vi "Compile Data Replays.vi"(6 "Channel Descriptors in":T1, 7 "LoopName":string, 8 "error in (no error)":errorcluster, 9 "Custom Device Ref":T8 format="%.0x", 11 "Data Replays Refs":T8[](array[typedef]) format="%.0x") -> (0 "error out":errorcluster, 1 "DataReplayVoltages":T9[](array[typedef]), 3 "Data Replays":T10[](array[typedef]), 4 "Channel Descriptors out":T1)   [LabVIEW 2011, in "Engine Sim System Explorer.lvlib"]
uses:
  Engine Sim System Explorer.lvlib
  Shared/DataReplayConfig.ctl
  <vilib>/NI Veristand/Custom Device API/Custom Device Item Ref.ctl
  Shared/DataReplayVoltageConfig.ctl
  Shared/Channel Descriptors.ctl
  Shared/FPGA Write Descriptor.ctl
  Shared/InputChannelTypes.ctl
  <vilib>/rvi/DataTransferAndStorage/Container/Common/niFpgaDataTypeControl.ctl
  Shared/FPGA Read Descriptor.ctl
  Shared/OutputChannelTypes.ctl
  Shared/Status Chan Descriptor.ctl
  TypeDefs/DataReplayCtrlStringInfo.ctl
  TypeDefs/FPGA Mem Size.ctl
  Shared/Engine Simulation Global.vi
  <vilib>/NI Veristand/Custom Device API/Get Item Property (I32).vi
  <vilib>/NI Veristand/Custom Device API/Get Item Property (Boolean).vi
  <vilib>/NI Veristand/Custom Device API/Get Item Property (Double).vi
  <vilib>/NI Veristand/Custom Device API/Get Item Property (U16).vi
  Engine Simulation Shared.lvlib
  <vilib>/NI Veristand/Custom Device API/Custom Device API.lvlib
  <userlib>/AES/RT/AES RT.lvlib
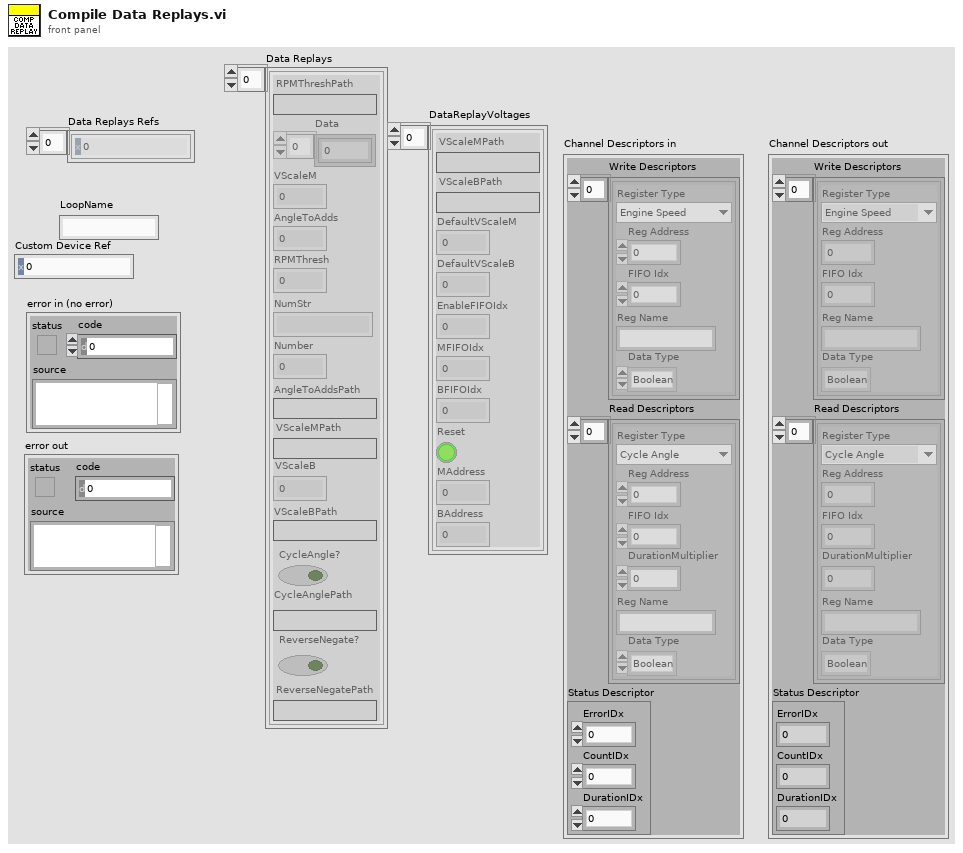
[diagram p1: front panel]
types:
  T1 = typedef "Engine Simulation Shared.lvlib/Channel Descriptors.ctl" = cluster{"Write Descriptors":T2[], "Read Descriptors":T5[], "Status Descriptor":T7}
  T2 = typedef "Engine Simulation Shared.lvlib/FPGA Write Descriptor.ctl" = cluster{"Register Type":T3, "Reg Address":u32, "FIFO Idx":i32, "Reg Name":string, "Data Type":T4}
  T3 = typedef "Engine Simulation Shared.lvlib/InputChannelTypes.ctl" = enum16{"Engine Speed", "Offset"}
  T4 = typedef "niFpgaDataTypeControl.ctl" = enum32{"Boolean", "I8", "I16", "I32", "I64", "U8", "U16", "U32", "U64", "FXP", "CustomControl"}
  T5 = typedef "Engine Simulation Shared.lvlib/FPGA Read Descriptor.ctl" = cluster{"Register Type":T6, "Reg Address":u32, "FIFO Idx":i32, "DurationMultiplier":dbl, "Reg Name":string, "Data Type":T4}
  T6 = typedef "Engine Simulation Shared.lvlib/OutputChannelTypes.ctl" = enum16{"Cycle Angle", "Crank Angle", "Time Duration", "Angle Duration", "Start Angle", "End Angle"}
  T7 = typedef "Engine Simulation Shared.lvlib/Status Chan Descriptor.ctl" = cluster{"ErrorIDx":i32, "CountIDx":i32, "DurationIDx":i32}
  T8 = typedef "Custom Device API.lvlib/Custom Device Item Ref.ctl" = u64
  T9 = typedef "Engine Simulation Shared.lvlib/DataReplayVoltageConfig.ctl" = cluster{"VScaleMPath":string, "VScaleBPath":string, "DefaultVScaleM":u32, "DefaultVScaleB":i32, "EnableFIFOIdx":i32, "MFIFOIdx":i32, "BFIFOIdx":i32, "Reset":bool, "MAddress":u32, "BAddress":u32}
  T10 = typedef "Engine Simulation Shared.lvlib/DataReplayConfig.ctl" = cluster{"RPMThreshPath":string, "Data":i16[], "VScaleM":u32, "AngleToAdds":u32, "RPMThresh":u64, "NumStr":string, "Number":i8, "AngleToAddsPath":string, "VScaleMPath":string, "VScaleB":i32, "VScaleBPath":string, "CycleAngle?":bool, "CycleAnglePath":string, "ReverseNegate?":bool, "ReverseNegatePath":string}
  T11 = typedef "Engine Sim System Explorer.lvlib/DataReplayCtrlStringInfo.ctl" = cluster{"LoopName":string, "ReplayName":string, "ReplayNumber":string}
  T12 = typedef "Engine Sim System Explorer.lvlib/FPGA Mem Size.ctl" = enum16{"32,768", "16,384", "8,192", "4,096", "2,048", "1024", "512", "256", "128"}
  T13 = typedef "Custom Device API.lvlib/Custom Device Item Info.ctl" = cluster{"Name":string, "Is Channel":bool, "GUID":string}
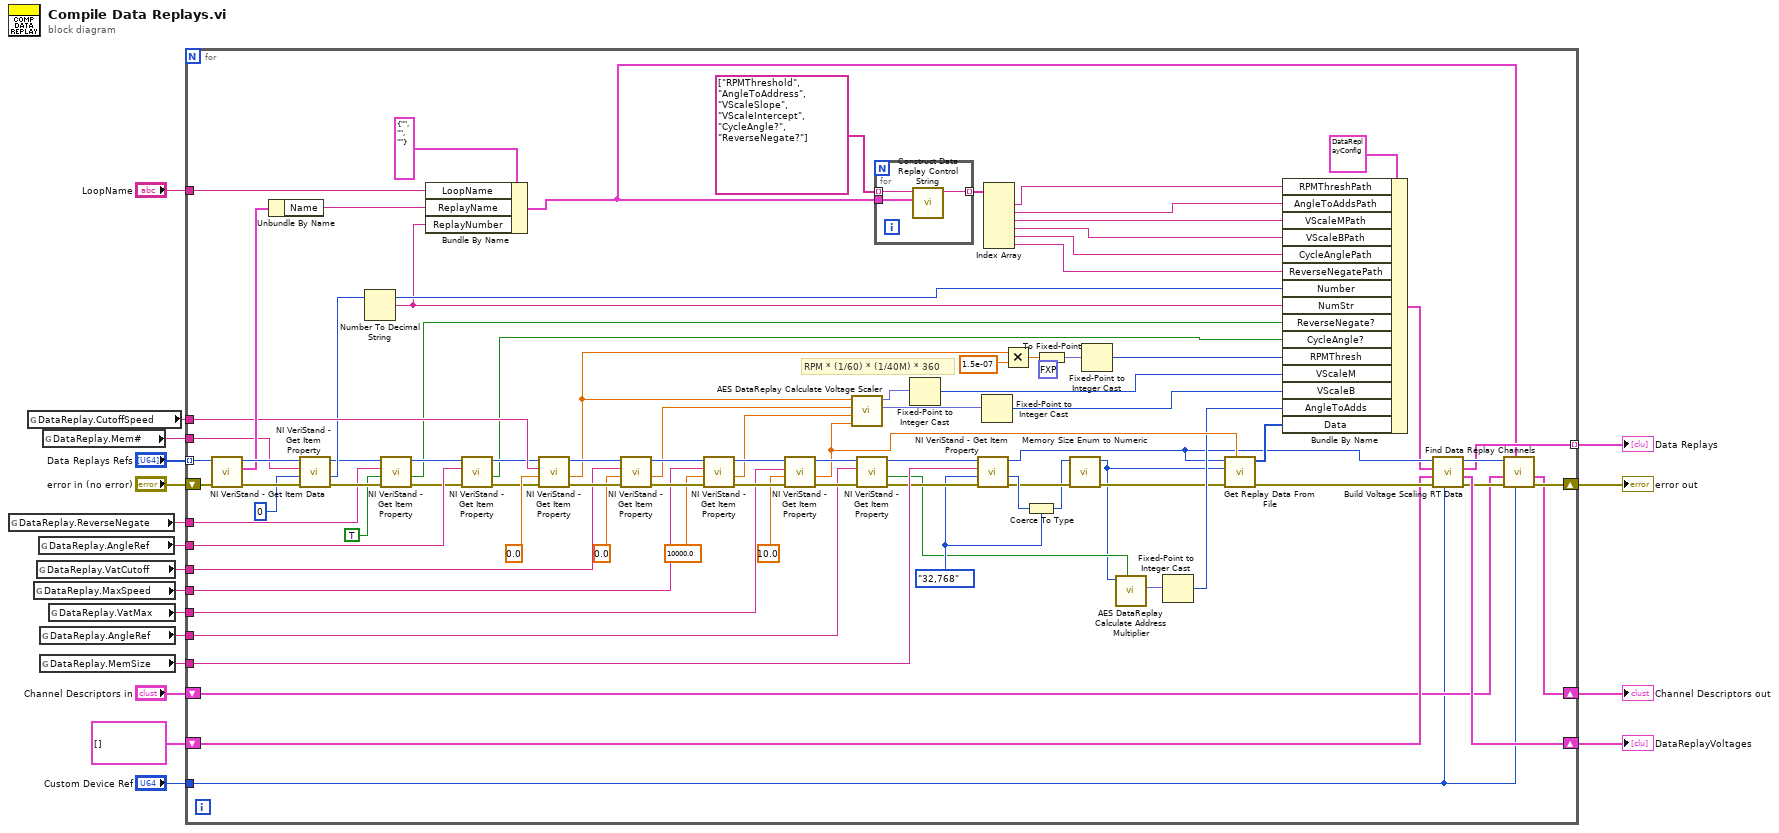
[diagram p0: block diagram]
diagram:
  n1 = global read "Engine Simulation Global.vi" "DataReplay.ReverseNegate"() -> (w6:string)
  n2 = global read "Engine Simulation Global.vi" "DataReplay.CutoffSpeed"() -> (w15:string)
  n3 = global read "Engine Simulation Global.vi" "DataReplay.MaxSpeed"() -> (w13:string)
  n4 = global read "Engine Simulation Global.vi" "DataReplay.VatCutoff"() -> (w14:string)
  n5 = global read "Engine Simulation Global.vi" "DataReplay.AngleRef"() -> (w7:string)
  n6 = global read "Engine Simulation Global.vi" "DataReplay.AngleRef"() -> (w11:string)
  n7 = global read "Engine Simulation Global.vi" "DataReplay.MemSize"() -> (w10:string)
  n8 = global read "Engine Simulation Global.vi" "DataReplay.Mem#"() -> (w16:string)
  n9 = global read "Engine Simulation Global.vi" "DataReplay.VatMax"() -> (w12:string)
  n10 = for {
    shift-right: [w30] -> w19
    shift-left: "error in (no error)" -> [w107]
    tunnel: "Data Replays Refs" -> [w104] mode=indexing
    tunnel: w16 -> [w101]
    tunnel: w15 -> [w92]
    tunnel: w14 -> [w91]
    tunnel: w13 -> [w90]
    tunnel: w12 -> [w89]
    tunnel: w11 -> [w80]
    tunnel: w10 -> [w78]
    tunnel: [w25] -> w9 mode=indexing
    tunnel: "LoopName" -> [w23]
    tunnel: w7 -> [w46]
    tunnel: w6 -> [w40]
    shift-right: [w35] -> w4
    shift-left: T9[] [] ("DataReplayVoltages") -> [w34]
    tunnel: "Custom Device Ref" -> [w26]
    shift-right: [w27] -> w1
    shift-left: "Channel Descriptors in" -> [w28]
    w62 = FPGA_Mem_Size."32,768" ("FPGA Memory Size")
    # "RPM * (1/60) * (1/40M) * 360"
    n11 = call <vilib>:"NI VeriStand - Get Item Data.vi"("error in (no error)"=w107, "Item Ref in"=w104) -> ("error out"=w105:errorcluster, "Item Info"=w102:T13, "Item Ref out"=w103:T8)  [unwired: 6 in, 1 out]
    n12 = Unbundle By Name(w102) -> ("Name"=w22:string)
    n13 = call-poly <vilib>:"NI VeriStand - Get Item Property.vi"("error in (no error)"=w105, "Default Value"=0, "Property Name"=w101, "Item Ref in"=w103) -> ("error out"=w96:errorcluster, "Value"=w68:i32, "Item Ref out"=w42:T8)  [unwired: 4 in, 1 out]
    n14 = Number To Decimal String(number=w68) -> (decimal integer string=w21:string)  [unwired: 1 in]
    n15 = call-poly <vilib>:"NI VeriStand - Get Item Property.vi"("error in (no error)"=w96, "Default Value"=TRUE, "Property Name"=w40, "Item Ref in"=w42) -> ("error out"=w43:errorcluster, "Value"=w38:bool, "Item Ref out"=w41:T8)  [unwired: 4 in, 1 out]
    n16 = Bundle By Name(cluster=T11 {"LoopName"="", "ReplayName"="", "ReplayNumber"=""} ("Control String Info"), "LoopName"=w23, "ReplayName"=w22, "ReplayNumber"=w21) -> (w20:T11)
    n17 = call-poly <vilib>:"NI VeriStand - Get Item Property.vi"("error in (no error)"=w43, "Property Name"=w46, "Item Ref in"=w41) -> ("error out"=w48:errorcluster, "Value"=w45:bool, "Item Ref out"=w47:T8)  [unwired: 5 in, 1 out]
    n18 = call-poly <vilib>:"NI VeriStand - Get Item Property.vi"("error in (no error)"=w48, "Default Value"=0.0, "Property Name"=w92, "Item Ref in"=w47) -> ("error out"=w95:errorcluster, "Value"=w71:dbl, "Item Ref out"=w99:T8)  [unwired: 4 in, 1 out]
    n19 = call-poly <vilib>:"NI VeriStand - Get Item Property.vi"("error in (no error)"=w95, "Default Value"=0.0, "Property Name"=w91, "Item Ref in"=w99) -> ("error out"=w94:errorcluster, "Value"=w84:dbl, "Item Ref out"=w98:T8)  [unwired: 4 in, 1 out]
    n20 = call-poly <vilib>:"NI VeriStand - Get Item Property.vi"("error in (no error)"=w94, "Default Value"=10000.0, "Property Name"=w90, "Item Ref in"=w98) -> ("error out"=w93:errorcluster, "Value"=w83:dbl, "Item Ref out"=w97:T8)  [unwired: 4 in, 1 out]
    n21 = call-poly <vilib>:"NI VeriStand - Get Item Property.vi"("error in (no error)"=w93, "Default Value"=10.0, "Property Name"=w89, "Item Ref in"=w97) -> ("error out"=w81:errorcluster, "Value"=w61:dbl, "Item Ref out"=w82:T8)  [unwired: 4 in, 1 out]
    n22 = call <userlib>:"AES DataReplay Calculate Voltage Scaler.vi"("maximum voltage"=w61, "maximum speed (RPM)"=w83, "threshold voltage"=w84, "threshold speed (RPM)"=w71) -> ("intercept (b)"=w58:fxp<+/-,18,3>, "slope (m)"=w59:fxp<+,18,12>)  [unwired: 6 in]
    n23 = call-poly <vilib>:"NI VeriStand - Get Item Property.vi"("error in (no error)"=w81, "Property Name"=w80, "Item Ref in"=w82) -> ("error out"=w77:errorcluster, "Value"=w53:bool, "Item Ref out"=w79:T8)  [unwired: 5 in, 1 out]
    n24 = for {
      tunnel: string[] ["RPMThreshold", "AngleToAddress", "VScaleSlope", "VScaleIntercept", "CycleAngle?", "ReverseNegate?"] -> [w110] mode=indexing
      tunnel: [w109] -> w67 mode=indexing
      tunnel: w20 -> [w108]
      n25 = call "Construct Data Replay Control String.vi"("Control String Info"=w108, "Control Name"=w110) -> ("Control"=w109:string)  [unwired: 9 in]
    }
    n26 = Fixed-Point to Integer Cast(1:w59) -> (0:w56:u32)
    n27 = call-poly <vilib>:"NI VeriStand - Get Item Property.vi"("error in (no error)"=w77, "Default Value"=w62, "Property Name"=w78, "Item Ref in"=w79) -> ("error out"=w55:errorcluster, "Value"=w76:u16, "Item Ref out"=w33:T8)  [unwired: 4 in, 1 out]
    n28 = Fixed-Point to Integer Cast(1:w58) -> (0:w57:i32)
    n29 = Index Array(array=w67) -> (element #1=w65:string, element #2=w64:string, element #3=w63:string, element #4=w60:string, element #5=w44:string, element #6=w37:string)  [unwired: 6 in]
    n30 = Multiply(x=w71, y=1.5e-07) -> (x*y=w74:dbl)
    n31 = Coerce To Type(0:w76, 1:w62) -> (2:w54:T12)
    n32 = To Fixed-Point(fixed-point type=fxp<+/-,47,-4> 0.0 ("Degrees/Tooth"), number=w74) -> (fixed-point=w72:fxp<+/-,47,-4>)
    n33 = call "Memory Size Enum to Numeric.vi"("error in (no error)"=w55, "FPGA Memory Size"=w54) -> ("error out"=w50:errorcluster, "Numeric"=w49:i32)  [unwired: 8 in]
    n34 = Fixed-Point to Integer Cast(1:w72) -> (0:w70:i64)
    n35 = call <userlib>:"AES DataReplay Calculate Address Multiplier.vi"("CycleAngle?"=w53, "memory size (divisible by 32)"=w49) -> ("angle to address multiplier"=w52:fxp<+,18,7>)  [unwired: 9 in]
    n36 = Fixed-Point to Integer Cast(1:w52) -> (0:w51:u32)
    n37 = call "Get Replay Data From File.vi"("V at Max RPM"=w61, "error in (no error)"=w50, "Memory Size (number)"=w49, "Item Ref in"=w33) -> ("error out"=w36:errorcluster, "DAC Data"=w69:i16[])  [unwired: 5 in, 1 out]
    n38 = Bundle By Name(cluster=T10 {"RPMThreshPath"="", "Data"=[], "VScaleM"=0, "AngleToAdds"=0, "RPMThresh"=0, "NumStr"="", "Number"=0, "AngleToAddsPath"="", "VScaleMPath"="", "VScaleB"=0, "VScaleBPath"="", "CycleAngle?"=FALSE, "CycleAnglePath"="", "ReverseNegate?"=FALSE, "ReverseNegatePath"=""} ("Profile Config"), "RPMThreshPath"=w65, "AngleToAddsPath"=w64, "VScaleMPath"=w63, "VScaleBPath"=w60, "CycleAnglePath"=w44, "ReverseNegatePath"=w37, "Number"=w68, "NumStr"=w21, "ReverseNegate?"=w38, "CycleAngle?"=w45, "RPMThresh"=w70, "VScaleM"=w56, "VScaleB"=w57, "AngleToAdds"=w51, "Data"=w69) -> (w32:T10)
    n39 = call "Build Voltage Scaling RT Data.vi"("Custom Device Ref"=w26, "error in (no error)"=w36, "DataReplayVoltages in"=w34, "DataReplay"=w32, "Replay ref in"=w33) -> ("error out"=w31:errorcluster, "DataReplayVoltages out"=w35:T9[], "DataReplay dup"=w25:T10, "Replay ref dup"=w29:T8)  [unwired: 3 in]
    n40 = call "Find Data Replay Channels.vi"("Custom Device Ref"=w26, "Control String Info"=w20, "error in (no error)"=w31, "Channel Descriptors in"=w28, "Replay ref"=w29) -> ("error out"=w30:errorcluster, "Channel Descriptors out"=w27:T1)  [unwired: 5 in]
  }
  "Data Replays" <- w9
  "error out" <- w19
  "DataReplayVoltages" <- w4
  "Channel Descriptors out" <- w1
